vi "sos_simple_2024.vi"(2 "xw H2O molar fraction":dbl, 3 "Temperature [K]":dbl=293.15, 4 "CO2 content (ppm)":dbl=500.0, 5 "Type of air":i32(listbox)=4) -> (0 "Simple speed of sound Zuck errata [m/s]":dbl format="%.4g", 1 "Simple speed of sound  correct [m/s]":dbl format="%.4g")   [LabVIEW 2016]
panel:
  out "rel. diff. (ppm)":dbl
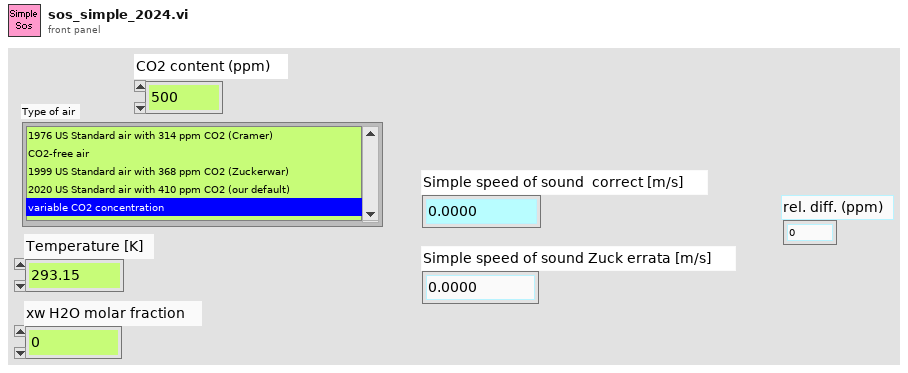
[diagram p1: front panel]
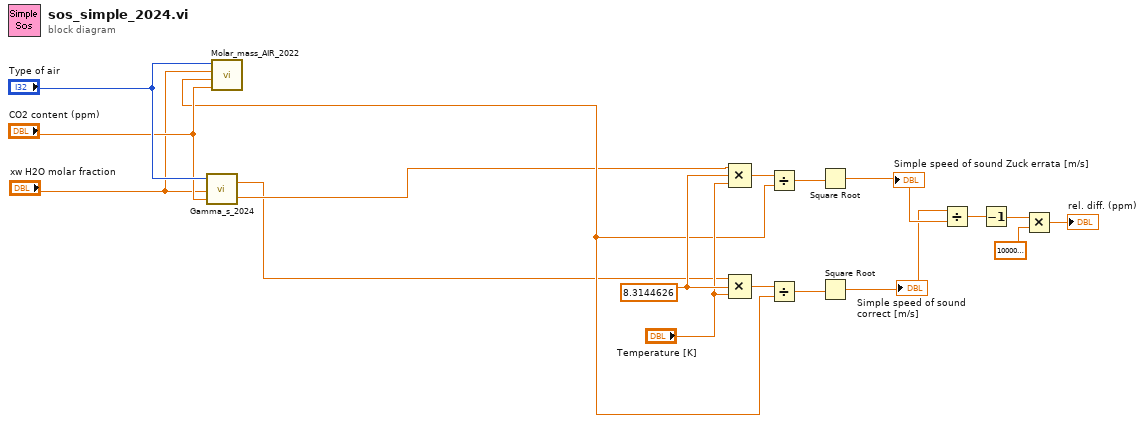
[diagram p0: block diagram]
diagram:
  w11 = 8.3144626
  n1 = call "Gamma_s_2024.vi"("CO2 content (ppm)"="CO2 content (ppm)", "xw molar fraction of water vapor"="xw H2O molar fraction", "Type of air"="Type of air") -> ("Gamma_s Zuckerwar (wrong)"=w8:dbl, "Gamma_s correct"=w7:dbl)
  n2 = call "Molar_mass_AIR_2022.vi"("CO2 content (ppm)"="CO2 content (ppm)", "xw molar fraction of water vapor"="xw H2O molar fraction", "Type of air"="Type of air") -> ("Molar mass humid air [kg/mol]"=w9:dbl)  [unwired: 8 out]
  n3 = Compound Arithmetic op=MULTIPLY(w8, w11, "Temperature [K]") -> (w13:dbl)
  n4 = Compound Arithmetic op=MULTIPLY(w7, w11, "Temperature [K]") -> (w18:dbl)
  n5 = Divide(x=w13, y=w9) -> (x/y=w12:dbl)
  n6 = Divide(x=w18, y=w9) -> (x/y=w17:dbl)
  n7 = Square Root(x=w12) -> (sqrt(x)=w5:dbl)
  "Simple speed of sound Zuck errata [m/s]" <- w5
  n8 = Square Root(x=w17) -> (sqrt(x)=w4:dbl)
  "Simple speed of sound  correct [m/s]" <- w4
  n9 = Divide(x=w4, y=w5) -> (x/y=w3:dbl)
  n10 = Decrement(x=w3) -> (x-1=w2:dbl)
  n11 = Multiply(x=w2, y=1000000.0) -> (x*y=→"rel. diff. (ppm)":dbl)
